vi "ADIS16448 Loop Cal Buffer.vi"(9 "Max Samples":i32=1, 10 "New Value":dbl, 11 "Cmd":T1) -> (3 "Mean":dbl)   [LabVIEW 2019]
uses:
  Typedef/ADIS16448 Call Buffer Cmd.ctl
  <vilib>/Analysis/baseanly.llb/Mean (DBL).vi
  <vilib>/Analysis/NI_AALBase.lvlib
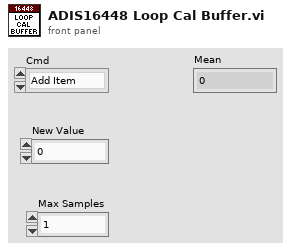
[diagram p1: front panel]
types:
  T1 = typedef "ADIS16448 Call Buffer Cmd.ctl" = enum16{"Add Item ", "Calculate"}
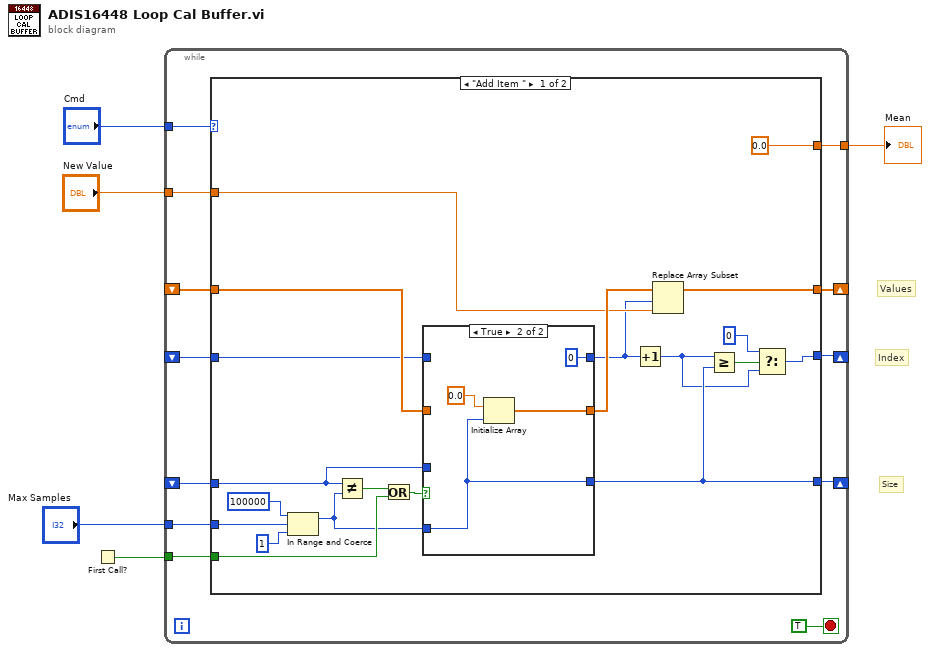
[diagram p0: block diagram]
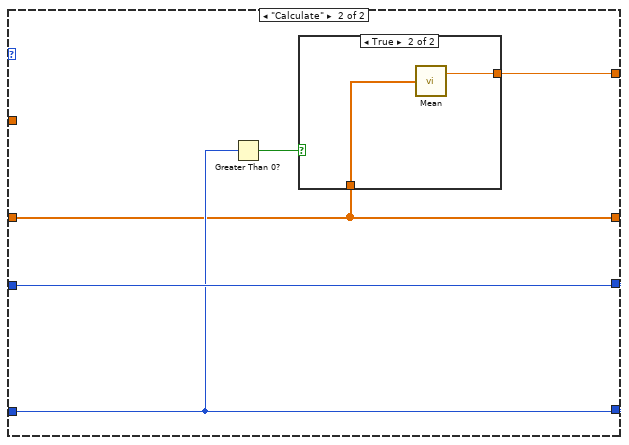
[diagram p3: hidden frame]
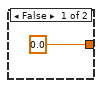
[diagram p4: hidden frame]
diagram:
  # "Values"
  # "Index"
  # "Size"
  n1 = First Call?() -> (First Call?: T/F=w4:bool)
  n2 = while {
    tunnel: "Cmd" -> [w17]
    shift-right: [w9] -> _
    shift-left: _ -> [w15]
    shift-right: [w8] -> _
    shift-left: _ -> [w13]
    tunnel: w4 -> [w14]
    shift-right: [w12] -> _
    shift-left: _ -> [w11]
    tunnel: "New Value" -> [w10]
    tunnel: [w7] -> w2
    tunnel: "Max Samples" -> [w6]
    stop <- TRUE stop-if-true
    n3 = case shown="\"Add Item \"" w17 {
      tunnel: w15 -> [w25 w48]
      tunnel: w14 -> [w36 _]
      tunnel: w13 -> [w24 w49]
      tunnel: [w33 w46] -> w12
      tunnel: w11 -> [w32 w46]
      tunnel: w10 -> [w31 _]
      tunnel: [w30 w48] -> w9
      tunnel: [w27 w49] -> w8
      tunnel: [0.0 ("mean") w45] -> w7
      tunnel: w6 -> [w18 _]
      frame "Add Item " {
        n4 = In Range and Coerce(upper limit=100000, x=w18, lower limit=1) -> (coerced(x)=w19:i32)  [unwired: 1 out]
        n5 = Not Equal?(x=w25, y=w19) -> (x != y?=w37:bool)
        n6 = Or(x=w37, y=w36) -> (x .or. y?=w35:bool)
        n7 = case shown="True" w35 {
          tunnel: w19 -> [_ w42]
          tunnel: [w40 w43] -> w34
          tunnel: w32 -> [w40 _]
          tunnel: [w39 w42] -> w30
          tunnel: w25 -> [w39 _]
          tunnel: w24 -> [w38 _]
          tunnel: [w38 0 ("t")] -> w23
          frame False {
          }
          frame True {
            n8 = Initialize Array(0.0 ("element"), w42) -> (w43:dbl[])
          }
        }
        n9 = Increment(x=w23) -> (x+1=w28:i32)
        n10 = Replace Array Subset(array=w34, new element=w31, index=w23) -> (w33:dbl[])
        n11 = Greater Or Equal?(x=w28, y=w30) -> (x >= y?=w29:bool)
        n12 = Select(t=0, s=w29, f=w28) -> (s? t:f=w27:i32)
      }
      frame "Calculate" {
        n13 = Greater Than 0?(x=w48) -> (x > 0?=w47:bool)
        n14 = case shown="True" w47 {
          tunnel: w46 -> [_ w52]
          tunnel: [0.0 ("mean") w51] -> w45
          frame False {
          }
          frame True {
            n15 = call-poly <vilib>:"Mean.vi"("X"=w52) -> ("mean"=w51:dbl)  [unwired: 1 out]
          }
        }
      }
    }
  }
  "Mean" <- w2
